vi "Constants info to String Arrays.vi"(11 "Constants Info":T1[](array[typedef])) -> (2 "Constant Info Results Str":string[][](array[string]), 3 "VI Names":string[](array[string]))   [LabVIEW 2019, in "Panther Dashboard.lvlib"]
uses:
  Panther Dashboard.lvlib
  Constant Info--cluster.ctl
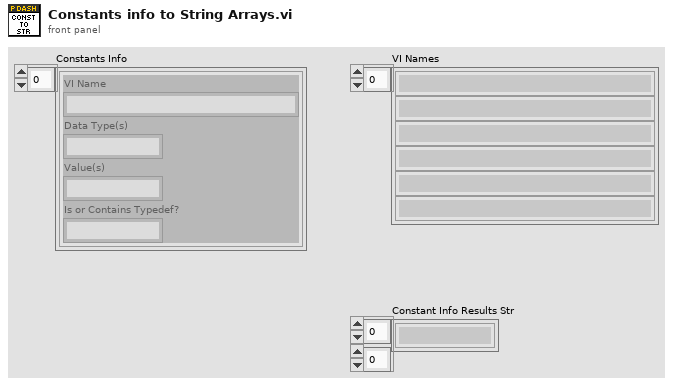
[diagram p1: front panel]
types:
  T1 = typedef "Panther Dashboard.lvlib/Constant Info--cluster.ctl" = cluster{"VI Name":string, "Data Type(s)":string, "Value(s)":string, "Is or Contains Typedef?":string}
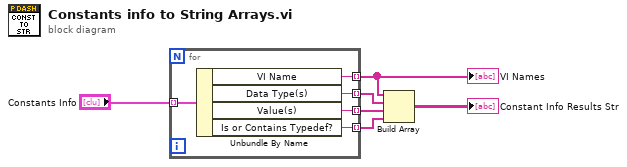
[diagram p0: block diagram]
diagram:
  n1 = for {
    tunnel: "Constants Info" -> [w11] mode=indexing
    tunnel: [w10] -> w5 mode=indexing
    tunnel: [w9] -> w4 mode=indexing
    tunnel: [w8] -> w3 mode=indexing
    tunnel: [w7] -> w2 mode=indexing
    n2 = Unbundle By Name(w11) -> ("VI Name"=w10:string, "Data Type(s)"=w9:string, "Value(s)"=w8:string, "Is or Contains Typedef?"=w7:string)
  }
  "VI Names" <- w5
  n3 = Build Array(w5, w4, w3, w2) -> (→"Constant Info Results Str":string[][])
